vi "User Table.vi"() -> ()   [LabVIEW 2019, in "User Lib.lvlib"]
uses:
  User Lib.lvlib
  <vilib>/Utility/miscctls.llb/LVRowAndColumnTypeDef.ctl
  <vilib>/addons/database/Connection.llb/DB Tools Open Connec (String).vi
  database.lvlib
  <vilib>/addons/database/NI_Database_API.lvlib
panel:
  in  "Cancel":bool
  in  "OK":bool
  in  "Error in 5":errorcluster
  out "Error out 5":errorcluster
  in  "Change Pass":bool
  out "data":string[][](array[string])
  in  "Error in 4":errorcluster
  out "Error out 4":errorcluster
  out "Error out 3":errorcluster
  in  "Error in 3":errorcluster
  in  "Error in 2":errorcluster
  out "Error out 2":errorcluster
  out "Error out":errorcluster
  in  "Error in":errorcluster
  in  "Delete":bool
  in  "Update":bool
  in  "New":bool
  out "User Table":string[][](table) caption="Thickness Table"
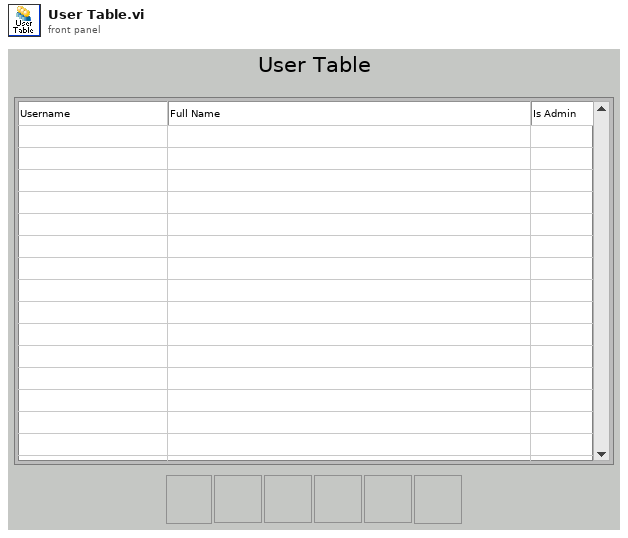
[diagram p1: front panel]
types:
  T1 = typedef "LVRowAndColumnTypeDef.ctl" = cluster{"Row":i32, "Column":i32}
  T2 = typedef "NI_Database_API.lvlib/Conn ObjectReference.ctl" = refnum<k1>
  T3 = cluster{i32, "date/time string":string, "date/time string":string, string}
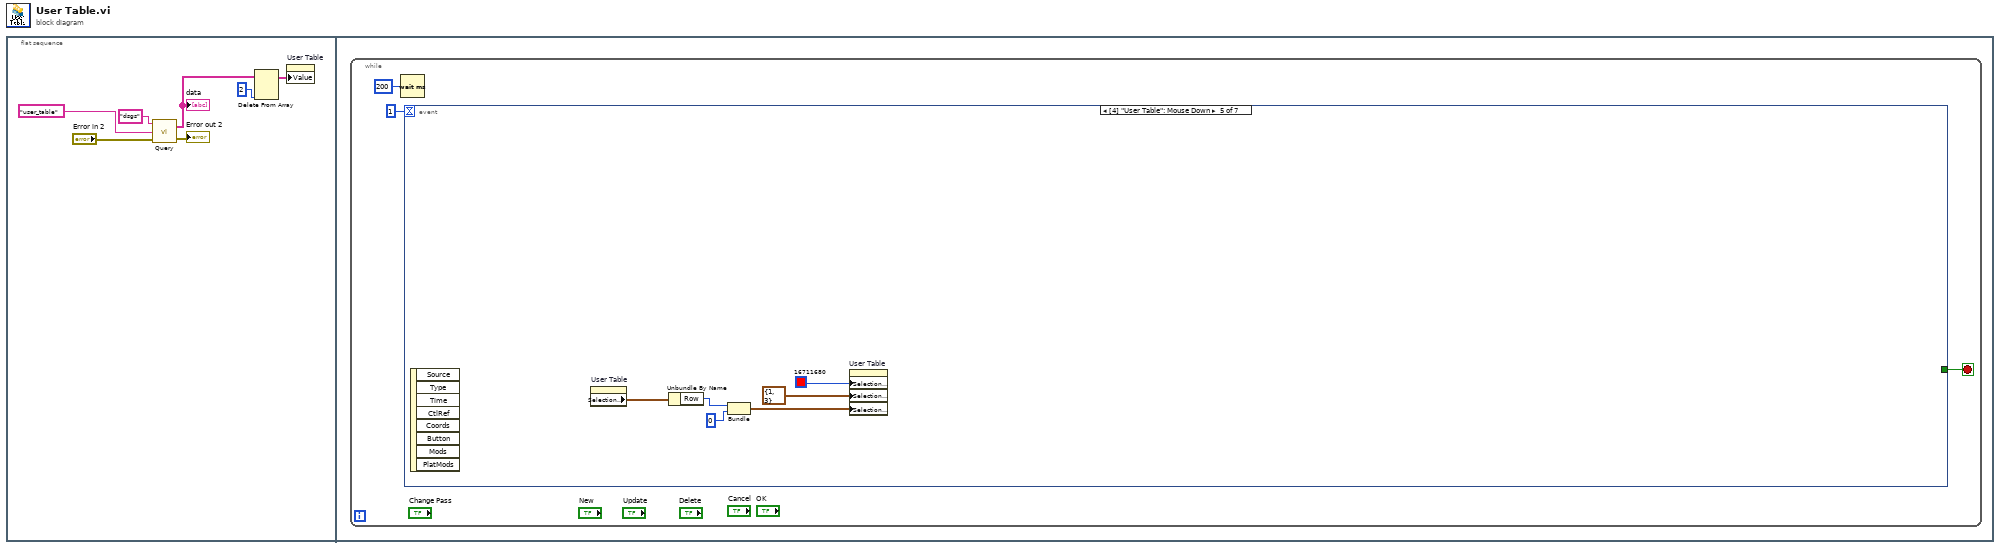
[diagram p0: block diagram]
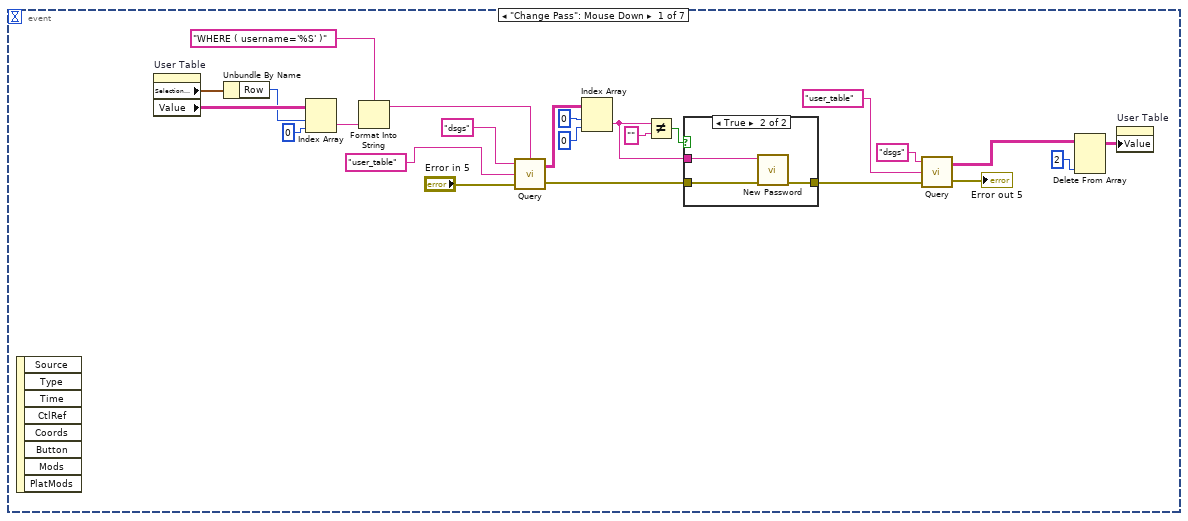
[diagram p2: hidden frame]
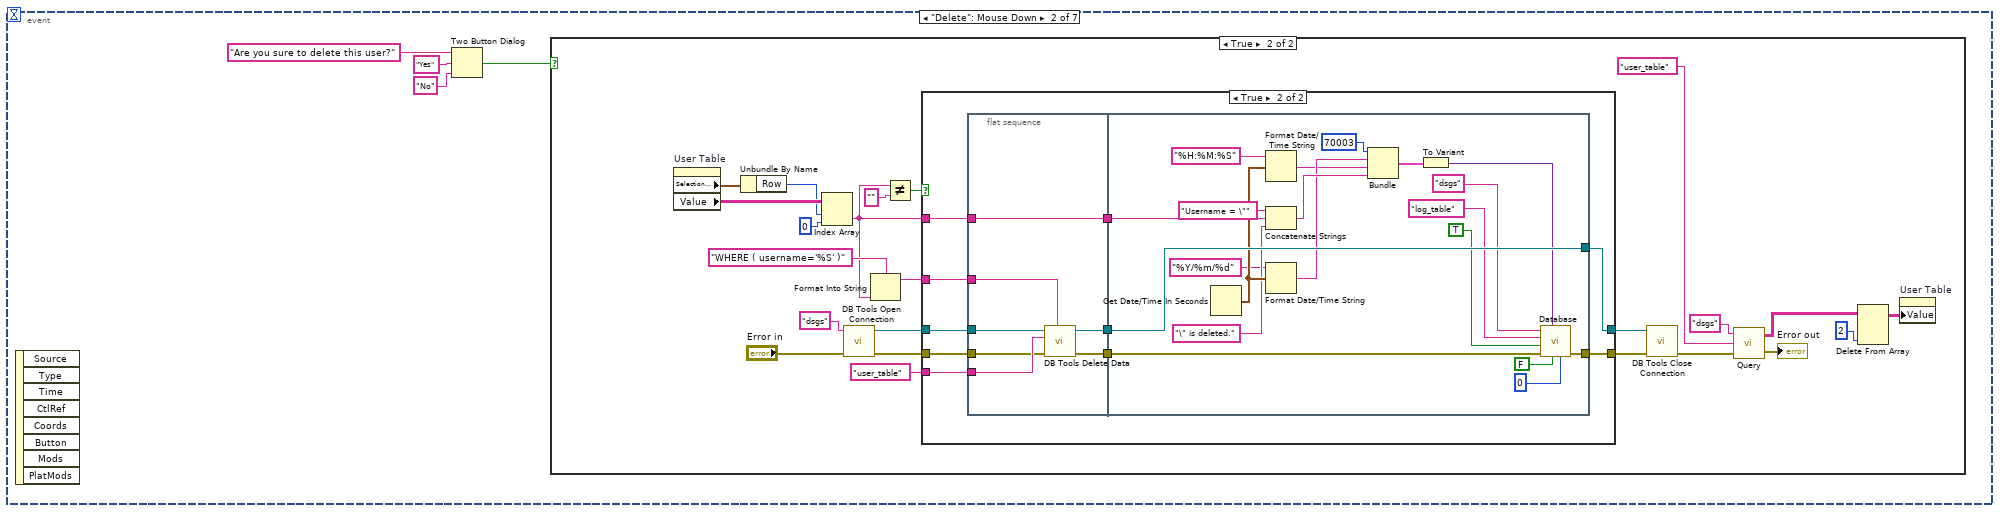
[diagram p4: hidden frame]
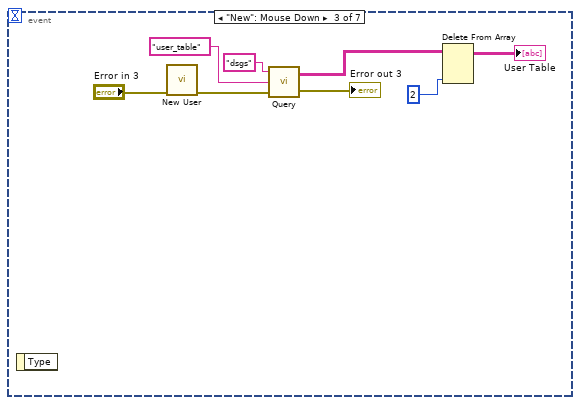
[diagram p7: hidden frame]
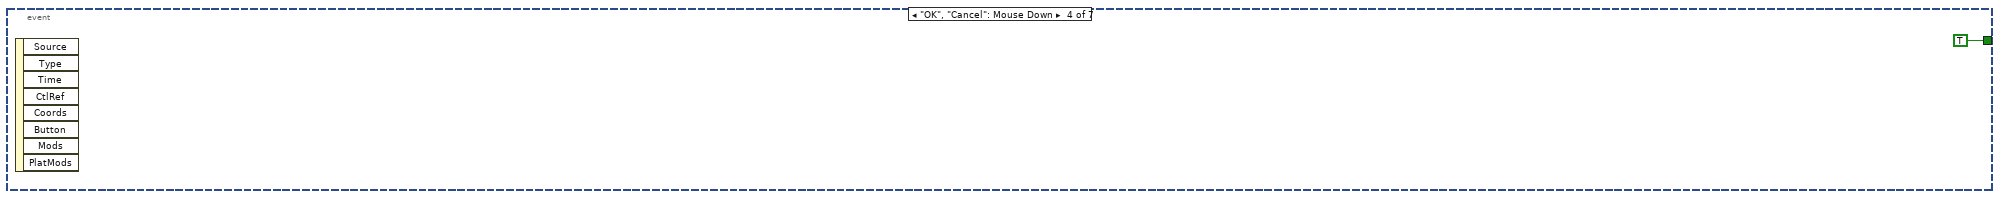
[diagram p8: hidden frame]
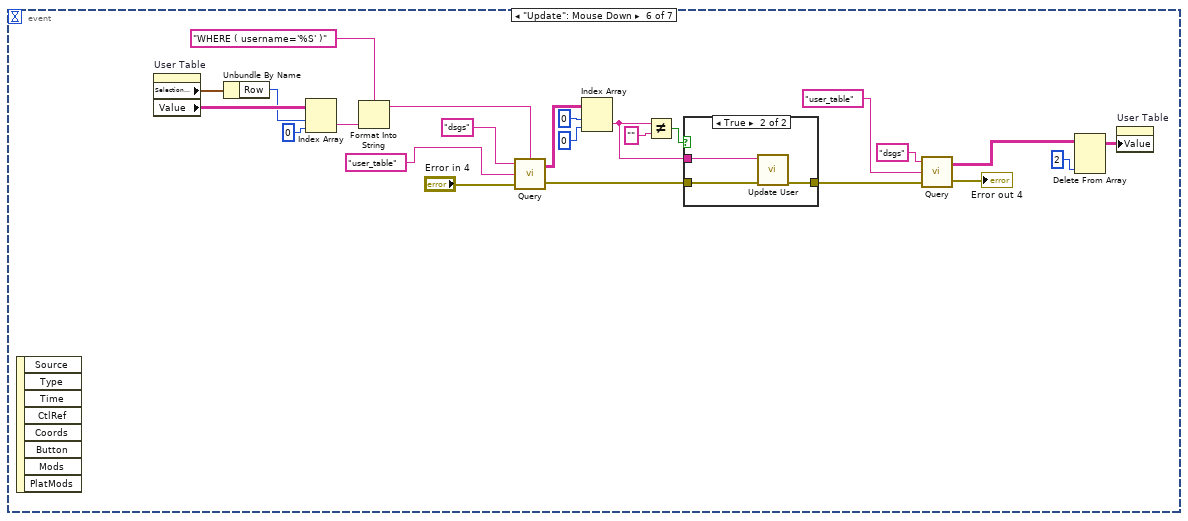
[diagram p9: hidden frame]
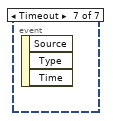
[diagram p11: hidden frame]
diagram:
  n1 = flat-sequence {
    frame #0 {
      n2 = call "Query.vi"("Error in"="Error in 2", "Table Name"="user_table", "Connection Name"="dsgs") -> ("Error out"=→"Error out 2":errorcluster, "data"=w4:string[][])  [unwired: 1 in]
      "data" <- w4
      n3 = Delete From Array(array=w4, index (col)=2 ("disabled index (col)")) -> (array with subset deleted=w3:string[][])  [unwired: 2 in, 1 out]
      n4 = property on="User Table" class="Tbl (strict)"("Value"=w3) -> ()  [unwired: 2 in, 2 out]
    }
    frame #1 {
      n5 = while {
        stop <- w8 stop-if-true
        n6 = Wait (ms)(milliseconds to wait=u32 200) -> ()  [unwired: 1 out]
        n7 = event shown="[4] \"User Table\": Mouse Down" {
          selector: _ -> [_ _ _ _ _ _ _]
          dyn-events: _ -> [_ _ _ _ _ _ _]
          timeout: 1 -> [_ _ _ _ _ _ _]
          tunnel: [_ _ _ TRUE _ _ _] -> w8
          event "Change Pass": Mouse Down {
            n8 = event-data() -> ()  [unwired: 1 in, 8 out]
            n9 = property on="User Table" class="Tbl (strict)"() -> ("Selection Start"=w32:T1, "Value"=w31:string[][])  [unwired: 2 in, 2 out]
            n10 = Unbundle By Name(w32) -> ("Row"=w30:i32)
            n11 = Index Array(array=w31, index (row)=w30, index (col)=0 ("disabled index (col)")) -> (element=w33:string)
            n12 = Format Into String(format string="WHERE ( username='%S' )" ("condition"), w33) -> (resulting string=w26:string)  [unwired: 2 in, 1 out]
            n13 = call "Query.vi"("Condition"=w26, "Error in"="Error in 5", "Table Name"="user_table", "Connection Name"="dsgs") -> ("Error out"=w27:errorcluster, "data"=w25:string[][])
            n14 = Index Array(array=w25, index (row)=0, index (col)=0 ("disabled index (col)")) -> (element=w24:string)
            n15 = Not Equal?(x=w24, y="") -> (x != y?=w23:bool)
            n16 = case shown="True" w23 {
              tunnel: [w35 w38] -> w29
              tunnel: w27 -> [w35 w37]
              tunnel: w24 -> [_ w36]
              frame False {
              }
              frame True {
                n17 = call "New Password.vi"("Error in"=w37, "Username"=w36) -> ("Error out"=w38:errorcluster)  [unwired: 9 in]
              }
            }
            n18 = call "Query.vi"("Error in"=w29, "Table Name"="user_table", "Connection Name"="dsgs") -> ("Error out"=→"Error out 5":errorcluster, "data"=w22:string[][])  [unwired: 1 in]
            n19 = Delete From Array(array=w22, index (col)=2 ("disabled index (col)")) -> (array with subset deleted=w21:string[][])  [unwired: 2 in, 1 out]
            n20 = property on="User Table" class="Tbl (strict)"("Value"=w21) -> ()  [unwired: 2 in, 2 out]
          }
          event "Delete": Mouse Down {
            n21 = event-data() -> ()  [unwired: 1 in, 8 out]
            n22 = Two Button Dialog(message="Are you sure to delete this user?", 1:"No" ("F button name (\"Cancel\")"), 2:"Yes" ("T button name (\"OK\")")) -> (T button?=w42:bool)
            n23 = case shown="True" w42 {
              frame False {
              }
              frame True {
                n24 = property on="User Table" class="Tbl (strict)"() -> ("Selection Start"=w65:T1, "Value"=w60:string[][])  [unwired: 2 in, 2 out]
                n25 = Unbundle By Name(w65) -> ("Row"=w59:i32)
                n26 = Index Array(array=w60, index (row)=w59, index (col)=0 ("disabled index (col)")) -> (element=w43:string)
                n27 = call-poly <vilib>:"DB Tools Open Connection.vi"("error in (no error)"="Error in", "connection information"="dsgs") -> ("error out"=w61:errorcluster, "connection reference"=w63:T2)  [unwired: 6 in]
                n28 = Format Into String(format string="WHERE ( username='%S' )" ("condition"), w43) -> (resulting string=w50:string)  [unwired: 2 in, 1 out]
                n29 = Not Equal?(x=w43, y="") -> (x != y?=w48:bool)
                n30 = case shown="True" w48 {
                  tunnel: w63 -> [w67 w77]
                  tunnel: "user_table" ("table") -> [_ w76]
                  tunnel: w61 -> [w66 w75]
                  tunnel: [w67 w74] -> w57
                  tunnel: [w66 w73] -> w56
                  tunnel: w50 -> [_ w72]
                  tunnel: w43 -> [_ w69]
                  frame False {
                  }
                  frame True {
                    n31 = flat-sequence {
                      tunnel: w77 -> [w84]
                      tunnel: w76 -> [w83]
                      tunnel: w75 -> [w82]
                      tunnel: w72 -> [w79]
                      tunnel: [w81] -> w71
                      tunnel: [w80] -> w70
                      tunnel: w69 -> [w78]
                      tunnel: [w78] -> w68
                      tunnel: [w87] -> w73
                      tunnel: [w104] -> w74
                      tunnel: w71 -> [w104]
                      tunnel: w70 -> [w88]
                      tunnel: w68 -> [w86]
                      frame #0 {
                        n32 = call <vilib>:"DB Tools Delete Data.vi"("condition"=w79, "error in (no error)"=w82, "table"=w83, "connection reference"=w84) -> ("error out"=w80:errorcluster, "connection reference out"=w81:T2)  [unwired: 6 in]
                      }
                      frame #1 {
                        n33 = Get Date/Time In Seconds() -> (seconds since 1Jan1904=w102:timestamp)
                        n34 = Format Date/Time String(time format string (%c)="%H:%M:%S", seconds (now)=w102) -> (date/time string=w100:string)  [unwired: 1 in]
                        n35 = Concatenate Strings("Username = \"" ("string"), w86, "\" is deleted." ("string")) -> (w103:string)
                        n36 = Format Date/Time String(time format string (%c)="%Y/%m/%d", seconds (now)=w102) -> (date/time string=w101:string)  [unwired: 1 in]
                        n37 = Bundle(70003, "date/time string"=w101, "date/time string"=w100, w103) -> (w99:T3)  [unwired: 1 in]
                        n38 = To Variant(anything=w99) -> (Variant=w98:variant)
                        n39 = call "Database.vi"("Maximum Row"=u64 0 ("Storage Time (Day)"), "Delete row?"=FALSE, "Data"=w98, "Error in"=w88, "Auto Increment ID?"=TRUE, "Table"="log_table" ("table"), "Connection"="dsgs" ("table")) -> ("Error out"=w87:errorcluster)  [unwired: 4 in]
                      }
                    }
                  }
                }
                n40 = call <vilib>:"DB Tools Close Connection.vi"("error in (no error)"=w56, "connection reference"=w57) -> ("error out"=w51:errorcluster)  [unwired: 5 in]
                n41 = call "Query.vi"("Error in"=w51, "Table Name"="user_table", "Connection Name"="dsgs") -> ("Error out"=→"Error out":errorcluster, "data"=w45:string[][])  [unwired: 1 in]
                n42 = Delete From Array(array=w45, index (col)=2 ("disabled index (col)")) -> (array with subset deleted=w44:string[][])  [unwired: 2 in, 1 out]
                n43 = property on="User Table" class="Tbl (strict)"("Value"=w44) -> ()  [unwired: 2 in, 2 out]
              }
            }
          }
          event "New": Mouse Down {
            n44 = event-data() -> ()  [unwired: 1 in, 1 out]
            n45 = call "New User.vi"("Error in"="Error in 3") -> ("Error out"=w108:errorcluster)  [unwired: 10 in]
            n46 = call "Query.vi"("Error in"=w108, "Table Name"="user_table", "Connection Name"="dsgs") -> ("Error out"=→"Error out 3":errorcluster, "data"=w107:string[][])  [unwired: 1 in]
            n47 = Delete From Array(array=w107, index (col)=2 ("disabled index (col)")) -> (array with subset deleted=→"User Table":string[][])  [unwired: 2 in, 1 out]
          }
          event "OK", "Cancel": Mouse Down {
            n48 = event-data() -> ()  [unwired: 1 in, 8 out]
          }
          event "User Table": Mouse Down {
            n49 = event-data() -> ()  [unwired: 1 in, 8 out]
            n50 = property on="User Table" class="Tbl (strict)"() -> ("Selection Start"=w116:T1)  [unwired: 2 in, 2 out]
            n51 = Unbundle By Name(w116) -> ("Row"=w117:i32)
            n52 = Bundle("Row"=w117, "Row"=0) -> (w119:cluster{"Row":i32, "Row":i32})  [unwired: 1 in]
            n53 = property on="User Table" class="Tbl (strict)"("Selection Color"=u32 16711680, "Selection Size"=T1 {"Row"=1, "Column"=3}, "Selection Start"=w119) -> ()  [unwired: 2 in, 2 out]
          }
          event "Update": Mouse Down {
            n54 = event-data() -> ()  [unwired: 1 in, 8 out]
            n55 = property on="User Table" class="Tbl (strict)"() -> ("Selection Start"=w143:T1, "Value"=w142:string[][])  [unwired: 2 in, 2 out]
            n56 = Unbundle By Name(w143) -> ("Row"=w141:i32)
            n57 = Index Array(array=w142, index (row)=w141, index (col)=0 ("disabled index (col)")) -> (element=w139:string)
            n58 = Format Into String(format string="WHERE ( username='%S' )" ("condition"), w139) -> (resulting string=w129:string)  [unwired: 2 in, 1 out]
            n59 = call "Query.vi"("Condition"=w129, "Error in"="Error in 4", "Table Name"="user_table", "Connection Name"="dsgs") -> ("Error out"=w130:errorcluster, "data"=w128:string[][])
            n60 = Index Array(array=w128, index (row)=0, index (col)=0 ("disabled index (col)")) -> (element=w125:string)
            n61 = Not Equal?(x=w125, y="") -> (x != y?=w124:bool)
            n62 = case shown="True" w124 {
              tunnel: [w144 w147] -> w134
              tunnel: w130 -> [w144 w146]
              tunnel: w125 -> [_ w145]
              frame False {
              }
              frame True {
                n63 = call "Update User.vi"("Error in"=w146, "Username"=w145) -> ("Error out"=w147:errorcluster)  [unwired: 9 in]
              }
            }
            n64 = call "Query.vi"("Error in"=w134, "Table Name"="user_table", "Connection Name"="dsgs") -> ("Error out"=→"Error out 4":errorcluster, "data"=w121:string[][])  [unwired: 1 in]
            n65 = Delete From Array(array=w121, index (col)=2 ("disabled index (col)")) -> (array with subset deleted=w120:string[][])  [unwired: 2 in, 1 out]
            n66 = property on="User Table" class="Tbl (strict)"("Value"=w120) -> ()  [unwired: 2 in, 2 out]
          }
          event Timeout {
            n67 = event-data() -> ()  [unwired: 1 in, 3 out]
          }
        }
      }
    }
  }
